vi "Request.vi"(0 "reference in":refnum<class "LoggerAdapter.lvclass">, 5 "Data":T1, 11 "Error In":errorcluster) -> (4 "reference out":refnum<class "LoggerAdapter.lvclass">, 15 "Error Out":errorcluster)   [LabVIEW 2024, in "LoggerAdapter.lvclass"]
doc: "Adapter request method"
uses:
  LoggerAdapter.lvclass
  Support/SignalData.ctl
  Support/LoggerData.ctl
  Logger_class/Logger.lvclass
  LoggerAdapter.lvclass/LoggerAdapter.ctl
panel:
  # "Connector Pane"
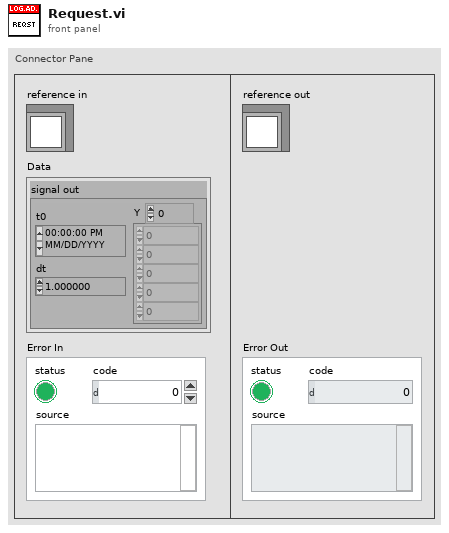
[diagram p1: front panel]
types:
  T1 = typedef "SignalData.ctl" = cluster{"signal out":waveform(dbl)}
  T2 = typedef "LoggerData.ctl" = cluster{"Signal Data":dbl[], "Timestamp Data":timestamp}
  T3 = typedef "LoggerAdapter.lvclass/ObjectAttributes.ctl" = cluster{"Adaptee":refnum<class "Logger.lvclass">}
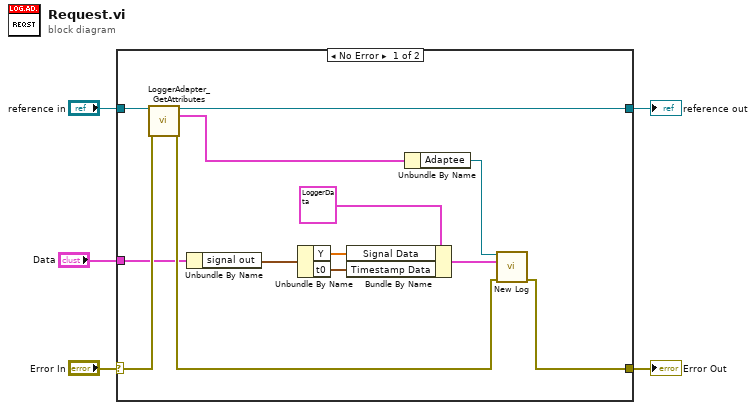
[diagram p0: block diagram]
diagram:
  n1 = case shown="No Error" "Error In" {
    selector: "Error In" -> [w18 w20]
    tunnel: [w13 w20] -> w4
    tunnel: [w15 w19] -> w2
    tunnel: "reference in" -> [w16 w19]
    tunnel: "Data" -> [w11 _]
    frame No Error {
      n2 = call "LoggerAdapter_GetAttributes.vi"("reference in"=w16, "Error In"=w18) -> ("reference out"=w15:refnum<class "LoggerAdapter.lvclass">, "Data"=w17:T3, "Error Out"=w14:errorcluster)  [unwired: 10 in, 1 out]
      n3 = Unbundle By Name(w11) -> ("signal out"=w10:waveform(dbl))
      n4 = Unbundle By Name(w10) -> ("Y"=w8:dbl[], "t0"=w7:timestamp)
      n5 = Bundle By Name(cluster=T2 {"Signal Data"=[], "Timestamp Data"=timestamp(0 s since 1904-01-01)} ("Logger Data"), "Signal Data"=w8, "Timestamp Data"=w7) -> (w6:T2)
      n6 = Unbundle By Name(w17) -> ("Adaptee"=w12:refnum<class "Logger.lvclass">)
      n7 = call-dynamic "New Log.vi"("reference in"=w12, "Logger Data"=w6, "Error In"=w14) -> ("Error Out"=w13:errorcluster)  [unwired: 11 in, 1 out]
    }
    frame Error {
    }
  }
  "Error Out" <- w4
  "reference out" <- w2
